vi "query_single_outlet.vi"(10 "outlet #":i32=1, 11 "IP / Hostname":string="172.20.125.112") -> (3 "status":bool)   [LabVIEW 2021]
panel:
  out "return code":i32
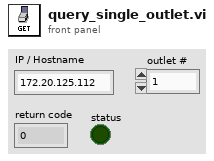
[diagram p1: front panel]
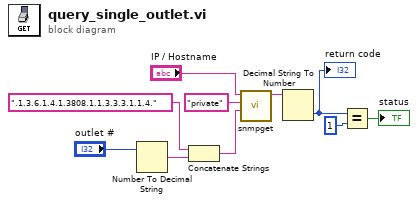
[diagram p0: block diagram]
diagram:
  n1 = Number To Decimal String(number="outlet #") -> (decimal integer string=w6:string)  [unwired: 1 in]
  n2 = Concatenate Strings(".1.3.6.1.4.1.3808.1.1.3.3.3.1.1.4." ("OID"), w6) -> (w5:string)
  n3 = call "snmpget.vi"("OID"=w5, "community"="private", "IP / Hostname"="IP / Hostname") -> ("return"=w3:string)  [unwired: 7 in, 1 out]
  n4 = Decimal String To Number(string=w3) -> (number=w10:i32)  [unwired: 2 in, 1 out]
  "return code" <- w10
  n5 = Equal?(x=w10, y=1) -> (x = y?=→"status":bool)
